vi "Set cif_waveformmonitor_Waveforms.vi"(7 "Complete Call (T)":bool=TRUE, 8 "error in (no error)":errorcluster, 10 "package_templatemessage":T1, 11 "gRPCid":T3) -> (0 "error out":errorcluster)   [LabVIEW 2021, in "CIFWaveformMonitor_server.lvlib"]
uses:
  CIFWaveformMonitor_server.lvlib
  <vilib>/gRPC/LabVIEW gRPC Library/Shared/grpcId.ctl
  cif_waveformmonitor_Waveforms.ctl
  cif_waveformmonitor_Waveform.ctl
  cif_waveformmonitor_Waveforms_Flat.ctl
  cif_waveformmonitor_Waveform_Flat.ctl
  dcc74a39-081a-4bdd-860b-8ed792803c96.vi
  RichToFlatcif_waveformmonitor_Waveform.vi
  <vilib>/gRPC/LabVIEW gRPC Library/Shared/TranslateGrpcError.vi
  <vilib>/gRPC/LabVIEW gRPC Library/Server API/Server/Get Server DLL Path.vi
  <vilib>/Utility/error.llb/Error Cluster From Error Code.vi
  <vilib>/gRPC/LabVIEW gRPC Library/grpc-lvsupport-release.lvlib
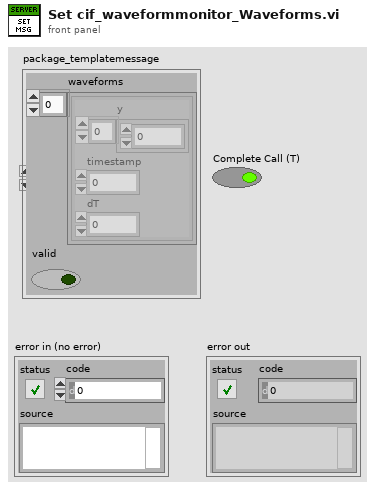
[diagram p1: front panel]
types:
  T1 = typedef "CIFWaveformMonitor_server.lvlib/cif_waveformmonitor_Waveforms.ctl" = cluster{"waveforms":T2[], "valid":bool}
  T2 = typedef "CIFWaveformMonitor_server.lvlib/cif_waveformmonitor_Waveform.ctl" = cluster{"y":dbl[], "timestamp":u64, "dT":dbl}
  T3 = typedef "grpc-lvsupport-release.lvlib/grpcId.ctl" = u64
  T4 = typedef "CIFWaveformMonitor_server.lvlib/cif_waveformmonitor_Waveforms_Flat.ctl" = cluster{"waveforms":T5[], "valid":bool}
  T5 = typedef "CIFWaveformMonitor_server.lvlib/cif_waveformmonitor_Waveform_Flat.ctl" = cluster{"y":dbl[], "timestamp":u64, "dT":dbl}
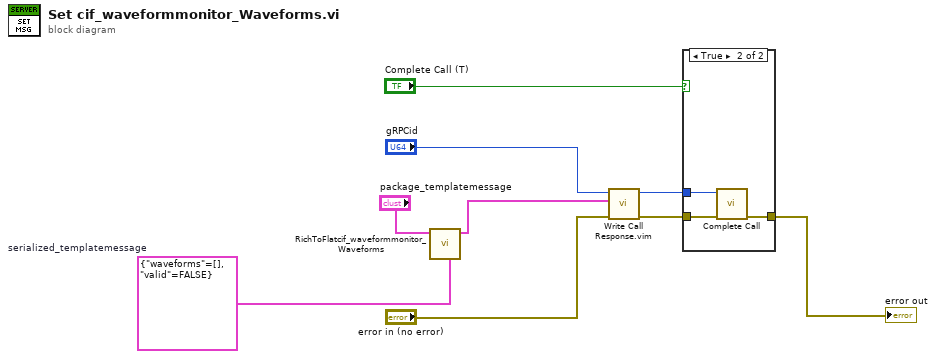
[diagram p0: block diagram]
diagram:
  w2 = T4 {"waveforms"=[], "valid"=FALSE}  # serialized_templatemessage
  n1 = call "RichToFlatcif_waveformmonitor_Waveforms.vi"("OutputClusterType"=w2, "InputCluster"="package_templatemessage") -> ("OutputCluster"=w1:T4)  [unwired: 9 in]
  n2 = call "Write Call Response.vim"("error in"="error in (no error)", "Response Data"=w1, "gRPCid in"="gRPCid") -> ("error out"=w6:errorcluster, "gRPCid out"=w7:T3)  [unwired: 7 in]
  n3 = case shown="True" "Complete Call (T)" {
    tunnel: [w10 w13] -> w9
    tunnel: w7 -> [_ w12]
    tunnel: w6 -> [w10 w11]
    frame False {
    }
    frame True {
      n4 = call <vilib>:"Complete Call.vi"("gRPCid"=w12, "error in"=w11) -> ("error out"=w13:errorcluster)  [unwired: 8 in]
    }
  }
  "error out" <- w9
